vi "zaber_readpos.vi"(8 "error in (no error)":errorcluster, 10 "axis":i32, 11 "VISA in":refnum<visa-resource-name>) -> (0 "error out":errorcluster, 2 "position":i32, 3 "VISA out":refnum<visa-resource-name>)   [LabVIEW 2020]
uses:
  ZaberTSeries.lvlib
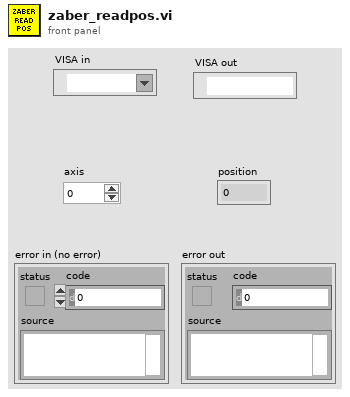
[diagram p1: front panel]
types:
  T1 = cluster{"axis":i32, "Command":u8, "Data":i32, "Response Count":i32}
  T2 = typedef "ZaberTSeries.lvlib/Response.ctl" = cluster{"Device Number":u8, "Command":u8, "Data":i32}
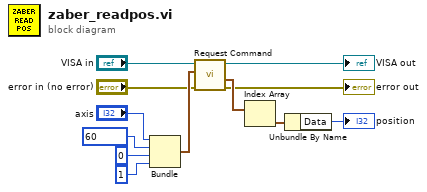
[diagram p0: block diagram]
diagram:
  w12 = u8 60 items=["Echo"=55, "Home"=1, "Move Absolute"=20, "Move Relative"=21, "Move at Constant Speed"=22, "Renumber"=2, "Restore Settings"=36, "Stop"=23] ("Command")
  n1 = Bundle("axis"="axis", "Command"=w12, "Data"=0, "Response Count"=1) -> (w9:T1)  [unwired: 1 in]
  n2 = call "Request Command.vi"("error in (no error)"="error in (no error)", "Request"=w9, "VISA resource name"="VISA in") -> ("error out"=→"error out":errorcluster, "Responses out"=w7:T2[], "VISA resource name out"=→"VISA out":refnum<visa-resource-name>)  [unwired: 5 in, 1 out]
  n3 = Index Array(array=w7) -> (element=w6:T2)  [unwired: 1 in]
  n4 = Unbundle By Name(w6) -> ("Data"=→"position":i32)
